vi "Multiple_DT98xx_Ain_PN.vi"(7 "Master board name":string="DT9816(00)", 8 "Samples per channel":u32=1000, 9 "Sampling rate (Hz)":dbl=20000.0, 10 "Slave channels to acquire":string="0,1,2,3,4,5", 11 "Master channels to acquire":string="0,1,2,3,4,5") -> (0 "Overall error":errorcluster, 2 "Slaves data":dbl[][][](array[numeric]), 3 "Master data":dbl[][](graph))   [LabVIEW 2011]
uses:
  <userlib>/LV-Link3/PolySubVIs/DtOLTimingSetInput.vi
  <userlib>/LV-Link3/PolySubVIs/DtCreateAinChan.vi
  <userlib>/LV-Link3/PolySubVIs/DtOLStartNormal.vi
  <userlib>/LV-Link3/PolySubVIs/DtCreateCtrRateChan.vi
  <userlib>/LV-Link3/PolySubVIs/DtOLReadMultiple2D.vi
panel:
  out "Slaves data (concat.)":dbl[][](graph)
  out "Master board index":i32
  out "Board names":string[](array[string])=["DT9816(00)", "DT9816(01)"]
  out "Number of boards":i32=2
  # "DEVICES MUST BE INTERCONNECTED AS FOLLOWS:\nMaster \"Counter 0 Out\" to Master \"Ext Clock\" and Slaves \"Ext Clock\""
  # "PN 18/10/2012"
  # "Device"
  # "Channel"
  # "Sample"
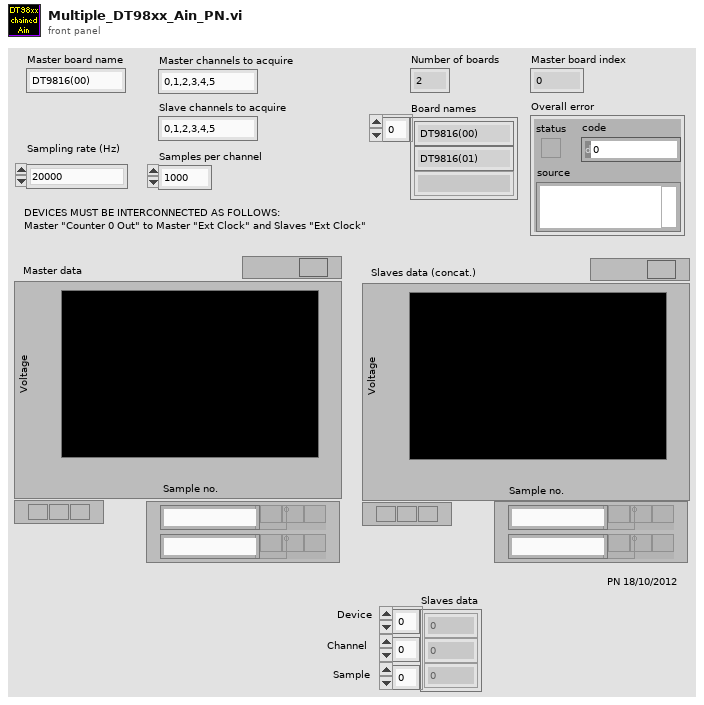
[diagram p1: front panel]
types:
  T1 = enum32{"Internal Clock", "External Clock", "No Timing"}
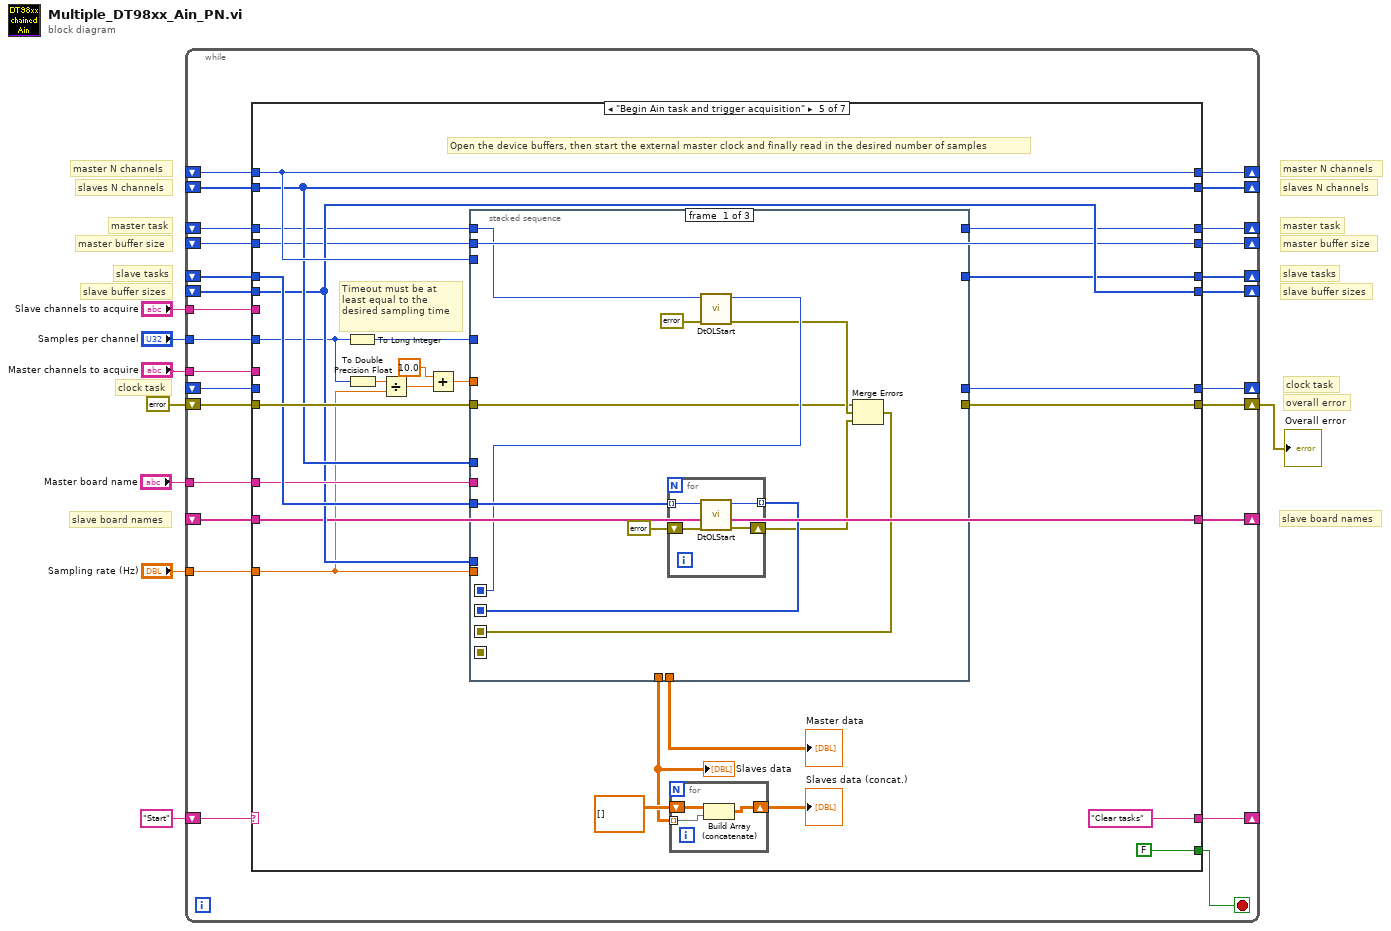
[diagram p0: block diagram]
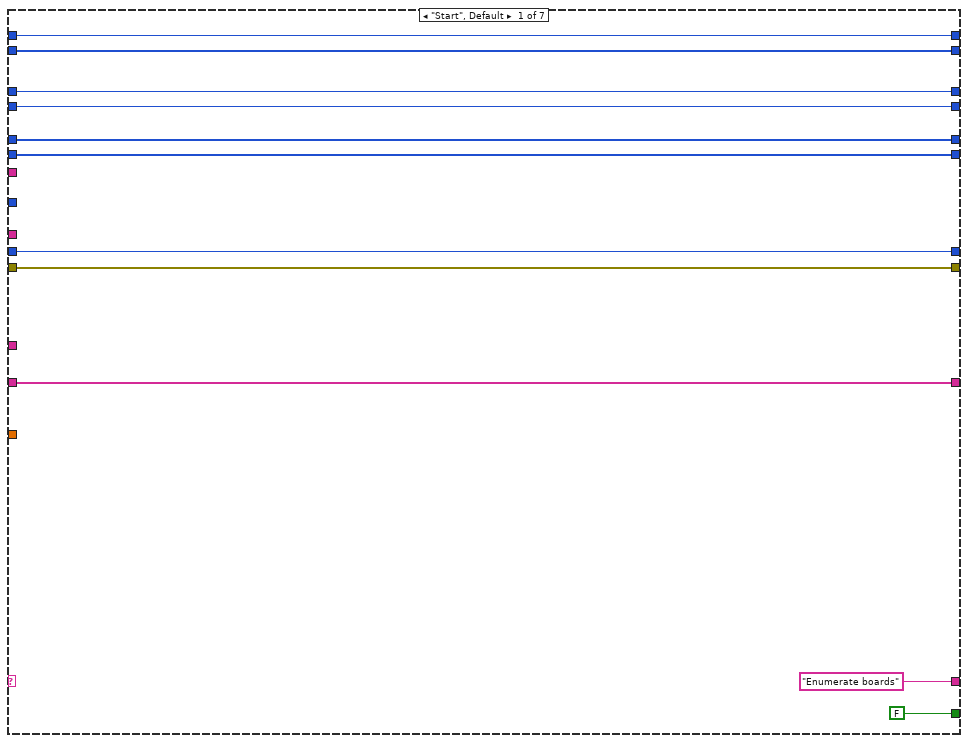
[diagram p2: hidden frame]
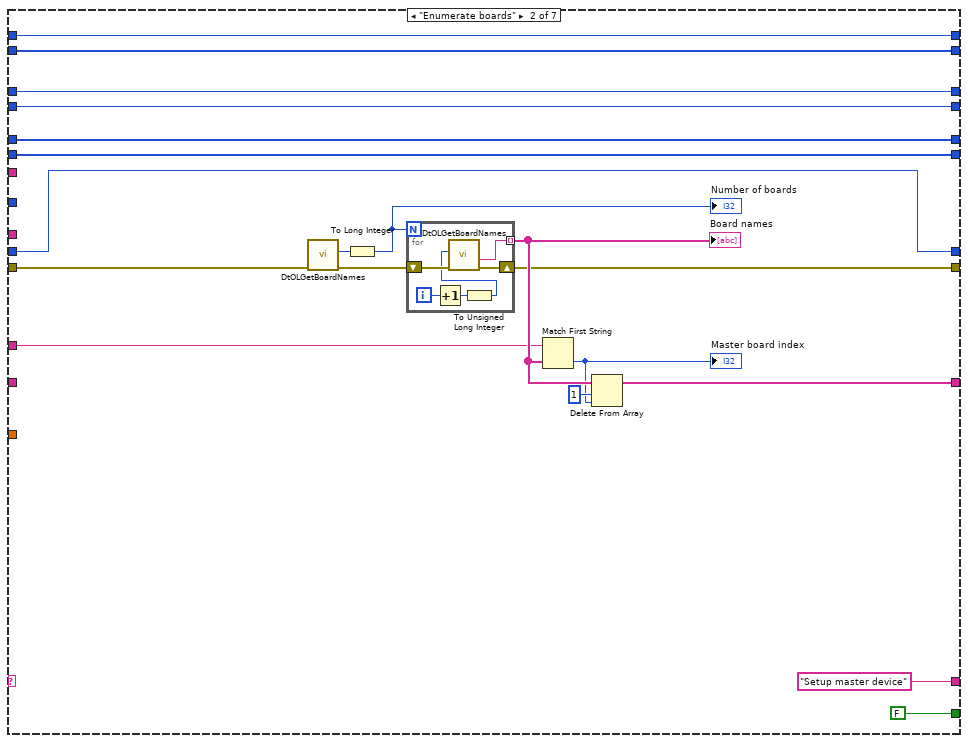
[diagram p3: hidden frame]
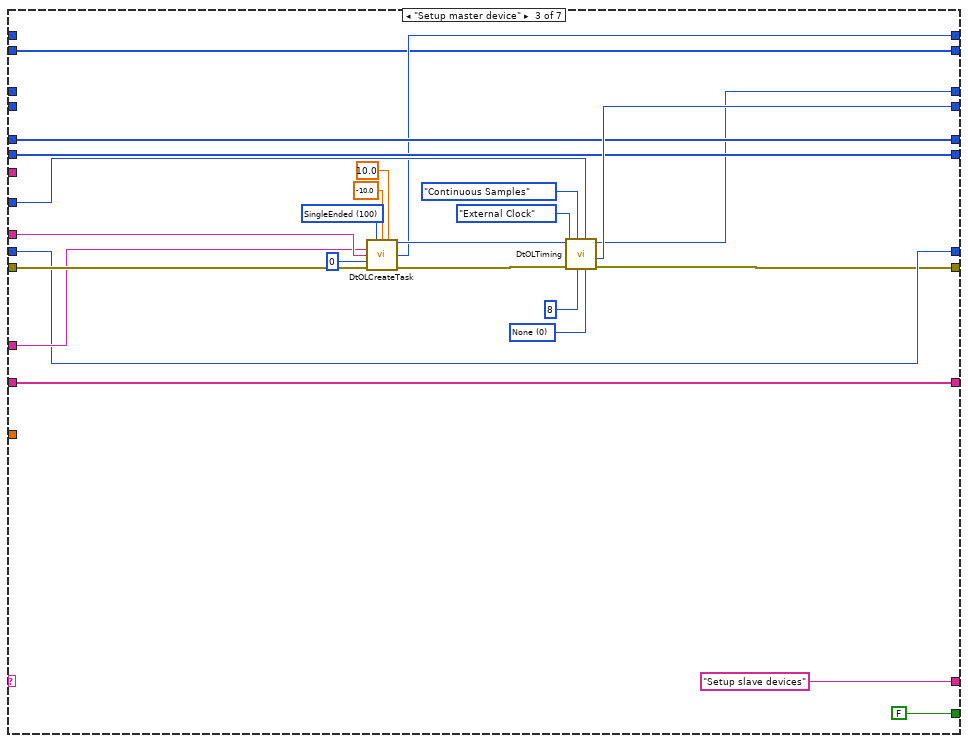
[diagram p4: hidden frame]
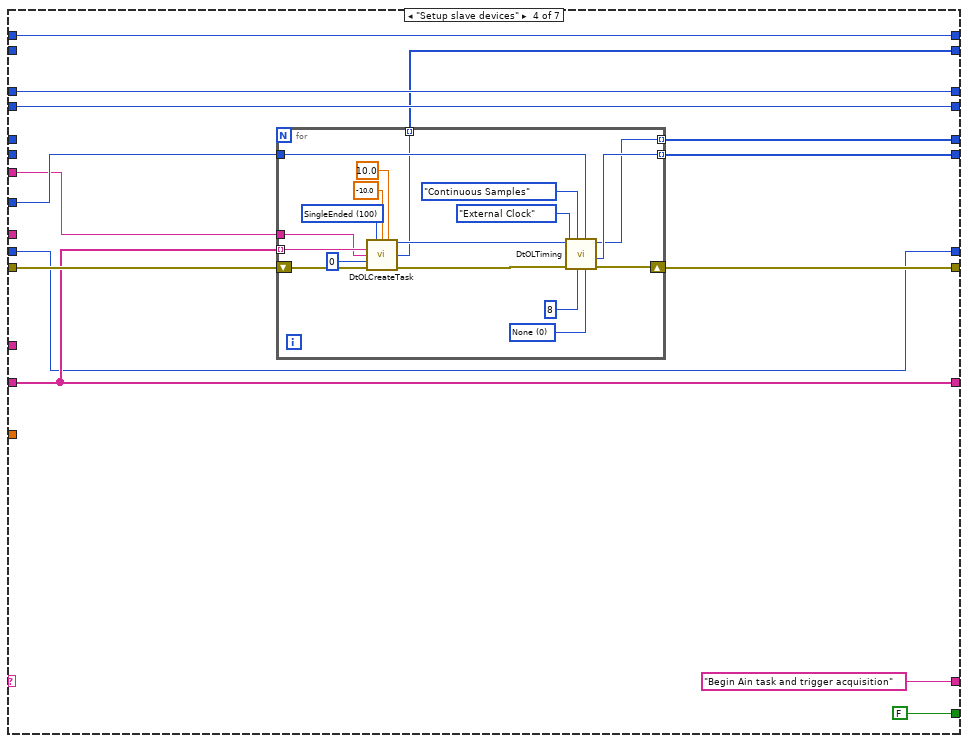
[diagram p5: hidden frame]
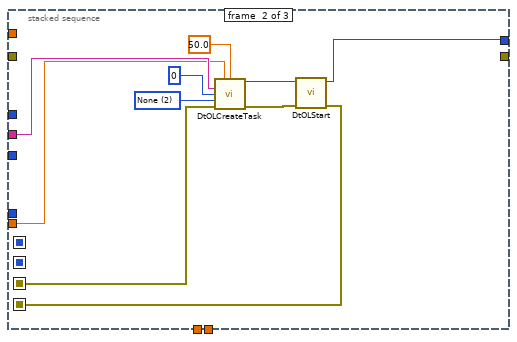
[diagram p6: hidden frame]
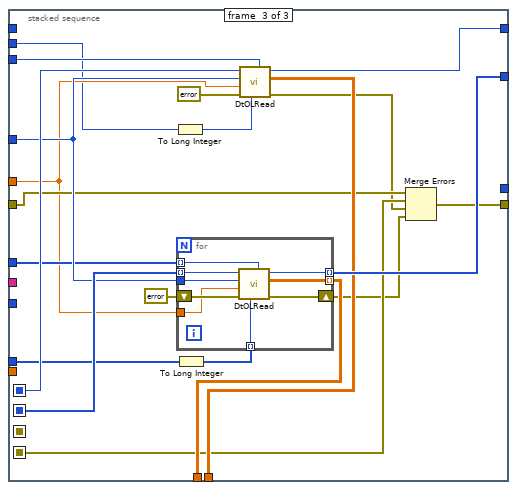
[diagram p7: hidden frame]
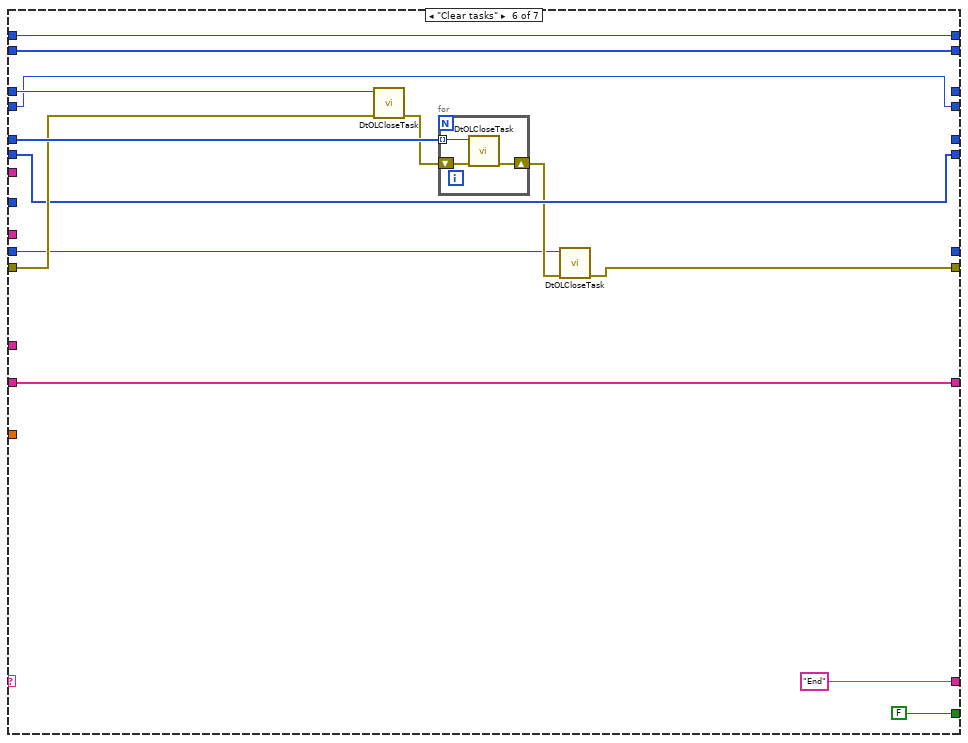
[diagram p8: hidden frame]
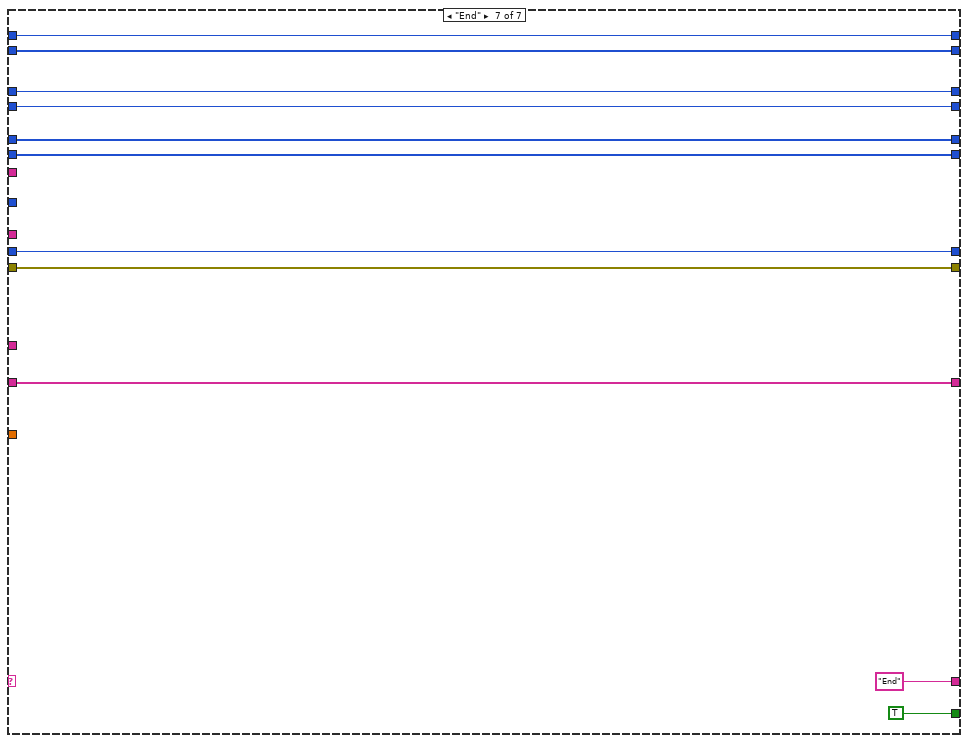
[diagram p9: hidden frame]
diagram:
  # "slave board names"
  # "clock task"
  # "slaves N channels"
  # "master N channels"
  # "master task"
  # "master buffer size"
  # "slave tasks"
  # "slave buffer sizes"
  # "overall error"
  # "clock task"
  # "slaves N channels"
  # "master N channels"
  # "master task"
  # "master buffer size"
  # "slave tasks"
  # "slave buffer sizes"
  # "slave board names"
  n1 = while {
    shift-right: [w32] -> _
    shift-left: "Start" -> [w33]
    shift-right: [w30] -> w1
    shift-left: errorcluster {"status"=FALSE, "code"=0, "source"=""} ("error in (no error)") -> [w31]
    shift-right: [w29] -> _
    shift-left: _ -> [w25]
    tunnel: "Master board name" -> [w28]
    tunnel: "Master channels to acquire" -> [w27]
    tunnel: "Samples per channel" -> [w26]
    shift-right: [w24] -> _
    shift-left: _ -> [w15]
    shift-right: [w23] -> _
    shift-left: _ -> [w14]
    shift-right: [w22] -> _
    shift-left: _ -> [w16]
    shift-right: [w21] -> _
    shift-left: _ -> [w17]
    shift-right: [w20] -> _
    shift-left: _ -> [w13]
    tunnel: "Sampling rate (Hz)" -> [w19]
    tunnel: "Slave channels to acquire" -> [w18]
    shift-right: [w12] -> _
    shift-left: _ -> [w9]
    shift-right: [w11] -> _
    shift-left: _ -> [w10]
    stop <- w34 stop-if-true
    n2 = case shown="\"Begin Ain task and trigger acquisition\"" w33 {
      tunnel: [FALSE FALSE FALSE FALSE FALSE FALSE TRUE] -> w34
      tunnel: ["Enumerate boards" "Setup master device" "Setup slave devices" "Begin Ain task and trigger acquisition" "Clear tasks" "End" "End"] -> w32
      tunnel: w31 -> [w38 w56 w81 w107 w151 w219 w229]
      tunnel: [w38 w55 w72 w106 w140 w212 w229] -> w30
      tunnel: [w37 w54 w78 w99 w143 w211 w228] -> w29
      tunnel: w28 -> [_ w53 w79 _ w149 _ _]
      tunnel: w27 -> [_ _ w80 _ _ _ _]
      tunnel: w26 -> [_ _ w83 w105 w136 _ _]
      tunnel: w25 -> [w37 _ w78 w99 w143 w211 w228]
      tunnel: [w41 w50 w76 w104 w129 _ w232] -> w24
      tunnel: [w40 w49 w75 w103 w146 w218 w231] -> w23
      tunnel: [w42 w51 w82 w100 w145 w217 w233] -> w22
      tunnel: [w43 w52 w71 w101 w130 _ w234] -> w21
      tunnel: [w39 w48 w77 w98 w137 _ w230] -> w20
      tunnel: w19 -> [_ _ _ _ w135 _ _]
      tunnel: w18 -> [_ _ _ w102 _ _ _]
      tunnel: w17 -> [w43 w52 _ w101 w144 w222 w234]
      tunnel: w16 -> [w42 w51 _ w100 w145 w217 w233]
      tunnel: w15 -> [w41 w50 w76 _ w150 w221 w232]
      tunnel: w14 -> [w40 w49 w75 _ w146 w218 w231]
      tunnel: w13 -> [w39 w48 w77 w98 _ w213 w230]
      tunnel: [w35 w46 w74 w96 w148 w216 w236] -> w12
      tunnel: [w36 w47 w73 w97 w147 w215 w235] -> w11
      tunnel: w10 -> [w36 w47 w73 _ w147 w215 w235]
      tunnel: w9 -> [w35 w46 _ w96 w148 w216 w236]
      frame "Start", Default {
      }
      frame "Enumerate boards" {
        n3 = call <userlib>:"DtOLGetBoardNames.vi"("error in (no error)"=w56) -> ("error out"=w60:errorcluster, "Number of boards"=w62:u32)  [unwired: 8 in, 1 out]
        n4 = To Long Integer(number=w62) -> (32bit integer=w61:i32)
        "Number of boards" <- w61
        n5 = for {
          N: w61 -> [_]
          shift-right: [w69] -> w55
          shift-left: w60 -> [w70]
          tunnel: [w68] -> w59 mode=indexing
          i -> [w67]
          n6 = Increment(x=w67) -> (x+1=w66:i32)
          n7 = To Unsigned Long Integer(number=w66) -> (unsigned 32bit integer=w65:u32)
          n8 = call <userlib>:"DtOLGetBoardNames.vi"("error in (no error)"=w70, "Select Board"=w65) -> ("error out"=w69:errorcluster, "Board Name"=w68:string)  [unwired: 7 in, 1 out]
        }
        "Board names" <- w59
        n9 = Match First String(2:w59, 3:w53) -> (0:w57:i32)  [unwired: 1 out]
        "Master board index" <- w57
        n10 = Delete From Array(array=w59, length=1, index=w57) -> (array with subset deleted=w54:string[])  [unwired: 1 out]
      }
      frame "Setup master device" {
        w84 = 0 items=["None", "Master", "Slave"] ("Sync Mode")
        w93 = 100 items=["SingleEnded"=100, "Differential"=101] ("Channel Type")
        n11 = call-poly <userlib>:"DtOLCreateTask.vi"("Channel Type"=w93, "Range Min"=-10.0, "Range Max"=10.0, "Board Name"=w79, "Channel"=w80, "Element"=u32 0, "error in (no error)"=w81) -> ("Task out"=w89:i32, "Actual Number of Channels"=w74:u32, "error out"=w88:errorcluster)  [unwired: 6 in]
        n12 = call-poly <userlib>:"DtOLTiming.vi"("Sync Mode"=w84, "Samples Per Channel"=w83, "Num Buffers"=u32 8, "Sample Mode"=enum16{"Finite Samples", "Continuous Samples"}."Continuous Samples", "error in (no error)"=w88, "Timing"=T1."External Clock", "Task in"=w89) -> ("error out"=w72:errorcluster, "Buffer Size"=w82:u32, "Task out"=w71:i32)  [unwired: 1 in, 1 out]
      }
      frame "Setup slave devices" {
        n13 = for {
          tunnel: w99 -> [w127] mode=indexing
          shift-right: [w110] -> w106
          shift-left: w107 -> [w125]
          tunnel: w102 -> [w123]
          tunnel: w105 -> [w116]
          tunnel: [w111] -> w104 mode=indexing
          tunnel: [w113] -> w103 mode=indexing
          tunnel: [w112] -> w97 mode=indexing
          w114 = 0 items=["None", "Master", "Slave"] ("Sync Mode")
          w126 = 100 items=["SingleEnded"=100, "Differential"=101] ("Channel Type")
          n14 = call-poly <userlib>:"DtOLCreateTask.vi"("Channel Type"=w126, "Range Min"=-10.0, "Range Max"=10.0, "Board Name"=w127, "Channel"=w123, "Element"=u32 0, "error in (no error)"=w125) -> ("Task out"=w120:i32, "Actual Number of Channels"=w112:u32, "error out"=w119:errorcluster)  [unwired: 6 in]
          n15 = call-poly <userlib>:"DtOLTiming.vi"("Sync Mode"=w114, "Samples Per Channel"=w116, "Num Buffers"=u32 8, "Sample Mode"=enum16{"Finite Samples", "Continuous Samples"}."Continuous Samples", "error in (no error)"=w119, "Timing"=T1."External Clock", "Task in"=w120) -> ("error out"=w110:errorcluster, "Buffer Size"=w113:u32, "Task out"=w111:i32)  [unwired: 1 in, 1 out]
        }
      }
      frame "Begin Ain task and trigger acquisition" {
        # "Timeout must be at least equal to the desired sampling time"
        # "Open the device buffers, then start the external master clock and finally read in the desired number of samples"
        n16 = To Long Integer(number=w136) -> (32bit integer=w128:i32)
        n17 = To Double Precision Float(number=w136) -> (double precision float=w134:dbl)
        n18 = Divide(x=w134, y=w135) -> (x/y=w132:dbl)
        n19 = Add(x=10.0, y=w132) -> (x+y=w133:dbl)
        n20 = stacked-sequence {
          seq-local: [w161 _ _] -> [_ _ w198]
          seq-local: [w160 _ _] -> [_ _ w197]
          seq-local: [w154 _ _] -> [_ w169 _]
          seq-local: [_ w168 _] -> [_ _ w187]
          tunnel: w151 -> [w155 _ w186]
          tunnel: w148 -> [_ _ w189]
          tunnel: w147 -> [_ _ w191]
          tunnel: w150 -> [w162 _ _]
          tunnel: w146 -> [_ _ w190]
          tunnel: w128 -> [_ _ w192]
          tunnel: w145 -> [_ _ w180]
          tunnel: w149 -> [_ w172 _]
          tunnel: w144 -> [w163 _ _]
          tunnel: [_ _ w183] -> w140
          tunnel: [_ _ w193] -> w139
          tunnel: [_ _ w194] -> w138
          tunnel: w135 -> [_ w171 _]
          tunnel: [_ w170 _] -> w137
          tunnel: w133 -> [_ _ w181]
          tunnel: [_ _ w196] -> w130
          tunnel: [_ _ w195] -> w129
          frame #0 {
            n21 = for {
              tunnel: w162 -> [w167] mode=indexing
              tunnel: [w166] -> w160 mode=indexing
              shift-right: [w164] -> w158
              shift-left: errorcluster {"status"=FALSE, "code"=0, "source"=""} ("error in (no error)") -> [w165]
              n22 = call-poly <userlib>:"DtOLStart.vi"("error in (no error)"=w165, "Task in"=w167) -> ("error out"=w164:errorcluster, "Task out"=w166:i32)  [unwired: 8 in]
            }
            n23 = call-poly <userlib>:"DtOLStart.vi"("error in (no error)"=errorcluster {"status"=FALSE, "code"=0, "source"=""}, "Task in"=w163) -> ("error out"=w159:errorcluster, "Task out"=w161:i32)  [unwired: 8 in]
            n24 = Merge Errors(w155, w159, w158) -> (w154:errorcluster)
          }
          frame #1 {
            w176 = 2 items=["LowLevel", "HighLevel", "None"] ("Gate Type")
            n25 = call-poly <userlib>:"DtOLCreateTask.vi"("Requested\nFrequency (Hz)"=w171, "Duty Cycle"=50.0, "Board Name"=w172, "Counter Num"=u32 0, "Gate Type"=w176, "error in (no error)"=w169) -> ("Task out"=w174:i32, "error out"=w173:errorcluster)  [unwired: 7 in, 1 out]
            n26 = call-poly <userlib>:"DtOLStart.vi"("error in (no error)"=w173, "Task in"=w174) -> ("error out"=w168:errorcluster, "Task out"=w170:i32)  [unwired: 8 in]
          }
          frame #2 {
            n27 = To Long Integer(number=w180) -> (32bit integer=w179:i32)
            n28 = To Long Integer(number=w190) -> (32bit integer=w178:i32[])
            n29 = for {
              tunnel: w197 -> [w207] mode=indexing
              tunnel: [w206] -> w195 mode=indexing
              tunnel: [w205] -> w193 mode=indexing
              tunnel: w192 -> [w204]
              tunnel: w191 -> [w203] mode=indexing
              tunnel: w178 -> [w202] mode=indexing
              shift-right: [w201] -> w184
              shift-left: errorcluster {"status"=FALSE, "code"=0, "source"=""} ("error in (no error)") -> [w200]
              tunnel: w181 -> [w199]
              n30 = call-poly <userlib>:"DtOLRead.vi"("Number Chan to Read"=w203, "Buffer size"=w202, "error in (no error)"=w200, "Timeout"=w199, "Samples Per Channel"=w204, "Task in"=w207) -> ("error out"=w201:errorcluster, "2D Data out"=w205:dbl[][], "Task out"=w206:i32)  [unwired: 1 in, 2 out]
            }
            n31 = call-poly <userlib>:"DtOLRead.vi"("Number Chan to Read"=w189, "Buffer size"=w179, "error in (no error)"=errorcluster {"status"=FALSE, "code"=0, "source"=""}, "Timeout"=w181, "Samples Per Channel"=w192, "Task in"=w198) -> ("error out"=w185:errorcluster, "2D Data out"=w194:dbl[][], "Task out"=w196:i32)  [unwired: 1 in, 2 out]
            n32 = Merge Errors(w186, w187, w185, w184) -> (w183:errorcluster)
          }
        }
        "Master data" <- w138
        "Slaves data" <- w139
        n33 = for {
          shift-right: [w210] -> w142
          shift-left: dbl[][] [] -> [w209]
          tunnel: w139 -> [w208] mode=indexing
          n34 = Build Array (concatenate)(w209, w208) -> (w210:dbl[][])
        }
        "Slaves data (concat.)" <- w142
      }
      frame "Clear tasks" {
        n35 = call <userlib>:"DtOLCloseTask.vi"("Error in"=w219, "Task in"=w222) -> ("Error Out"=w220:errorcluster)  [unwired: 9 in]
        n36 = for {
          tunnel: w221 -> [w227] mode=indexing
          shift-right: [w225] -> w214
          shift-left: w220 -> [w226]
          n37 = call <userlib>:"DtOLCloseTask.vi"("Error in"=w226, "Task in"=w227) -> ("Error Out"=w225:errorcluster)  [unwired: 9 in]
        }
        n38 = call <userlib>:"DtOLCloseTask.vi"("Error in"=w214, "Task in"=w213) -> ("Error Out"=w212:errorcluster)  [unwired: 9 in]
      }
      frame "End" {
      }
    }
  }
  "Overall error" <- w1
